vi "Roll Process.vi"() -> ()   [LabVIEW 2009]
uses:
  <vilib>/Utility/file.llb/Read From Spreadsheet File (string).vi
  <vilib>/Utility/file.llb/Write To Spreadsheet File (string).vi
panel:
  out "P 4":string[](array[string])
  out "P 3":string[](array[string])
  out "P 2":string[](array[string])
  out "P 1":string[](array[string])
  out "L 4":string[](array[string])
  out "L 3":string[](array[string])
  out "L 2":string[](array[string])
  out "L 1":string[](array[string])
  out "Cool Down Laps":string[](array[string])
  out "Warm Up Laps":string[](array[string])
  out "Cycle":string[](array[string])
  out "Length":string[](array[string])
  out "Chamber":string[](array[string])
  out "Value":string[][](array[string])
  in  "New Recipe":bool
  in  "Recipe Name":string
  in  "Save Recipe File":bool
  in  "Load Recipe File":bool
  in  "Recipe Table":string[][](table)
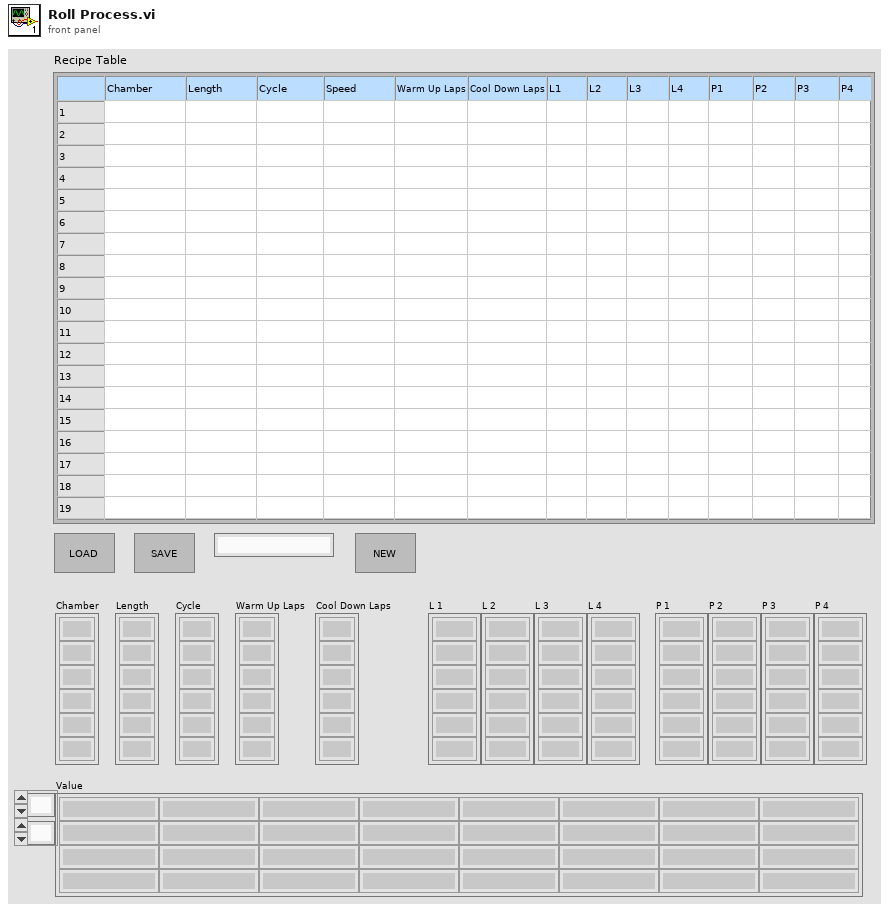
[diagram p1: front panel]
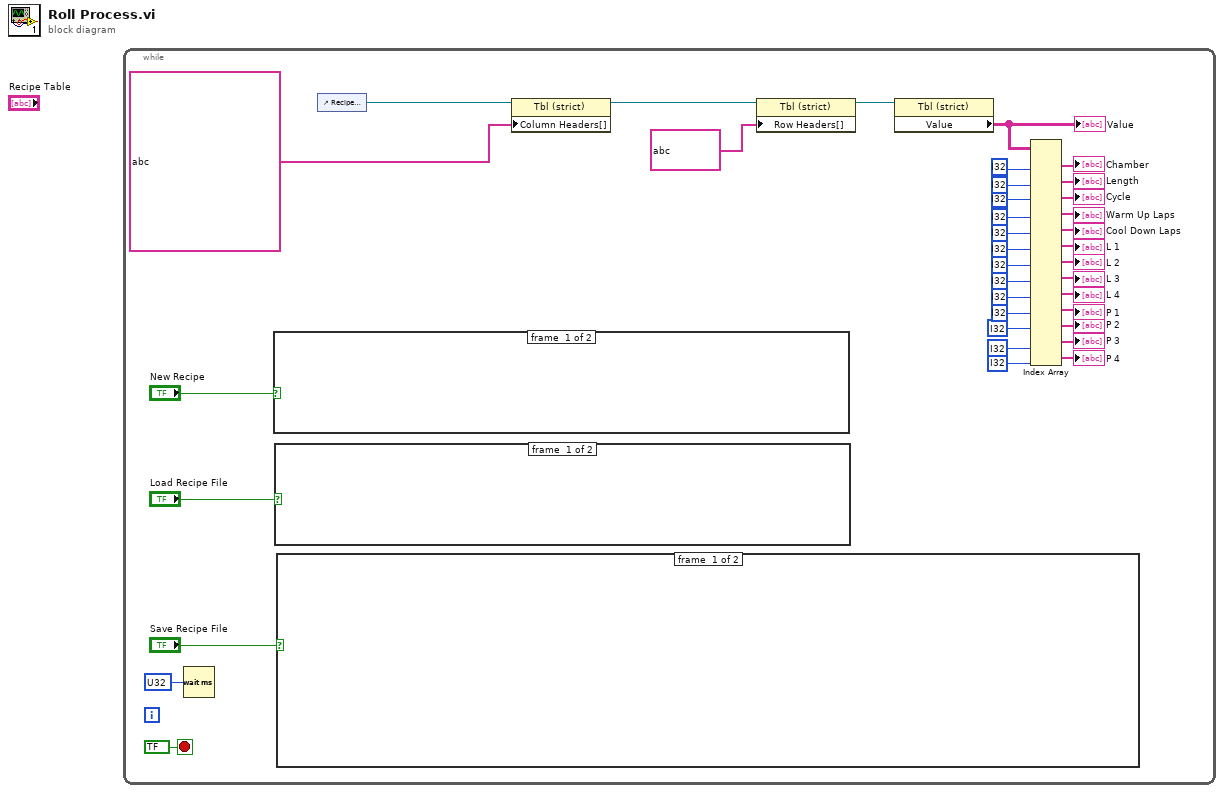
[diagram p0: block diagram]
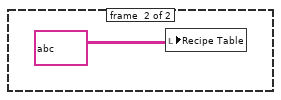
[diagram p2: hidden frame]
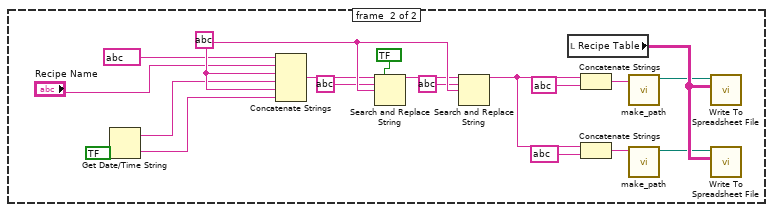
[diagram p3: hidden frame]
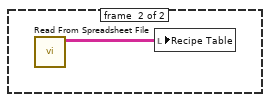
[diagram p4: hidden frame]
diagram:
  n1 = while {
    stop <- bool ? stop-if-true
    n2 = Wait (ms)(milliseconds to wait=u32 ?) -> ()  [unwired: 1 out]
    n3 = case shown="True" "New Recipe" {
      frame #0 {
      }
      frame #1 {
        n4 = local write "Recipe Table"(string[][] ? ("Row Header Strings[]")) -> ()
      }
    }
    n5 = case shown="True" "Load Recipe File" {
      frame #0 {
      }
      frame #1 {
        n6 = call-poly <vilib>:"Read From Spreadsheet File.vi"() -> ("all rows"=w58:string[][])  [unwired: 7 in, 4 out]
        n7 = local write "Recipe Table"(w58) -> ()
      }
    }
    n8 = case shown="True" "Save Recipe File" {
      frame #0 {
      }
      frame #1 {
        w49 = string ? ("string")
        n9 = Get Date/Time String(want seconds? (F)=bool ?) -> (date string=w42:string, time string=w43:string)  [unwired: 2 in]
        n10 = Concatenate Strings(string ? ("file_name"), "Recipe Name", w49, w42, w49, w43) -> (w44:string)
        n11 = Search and Replace String(replace all?=bool ? ("replace all? (F)"), input string=w44, search string=string ?, replace string=w49) -> (result string=w47:string)  [unwired: 4 in, 3 out]
        n12 = Search and Replace String(input string=w47, search string=string ?, replace string=w49) -> (result string=w51:string)  [unwired: 5 in, 3 out]
        n13 = local read "Recipe Table"() -> (w57:string[][])
        n14 = Concatenate Strings(w51, string ? ("string")) -> (w53:string)
        n15 = Concatenate Strings(w51, string ? ("string")) -> (w54:string)
        n16 = call "make_path.vi"("file_name"=w53) -> ("file path"=w55:path)  [unwired: 10 in]
        n17 = call "make_path.vi"("file_name"=w54) -> ("file path"=w56:path)  [unwired: 10 in]
        n18 = call-poly <vilib>:"Write To Spreadsheet File.vi"("2D data"=w57, "file path (dialog if empty)"=w55) -> ()  [unwired: 6 in, 1 out]
        n19 = call-poly <vilib>:"Write To Spreadsheet File.vi"("2D data"=w57, "file path (dialog if empty)"=w56) -> ()  [unwired: 6 in, 1 out]
      }
    }
    n20 = control-ref of="Recipe Table"() -> (w29:refnum<vi>)
    n21 = property class="Tbl (strict)"(reference=w29, "Column Headers[]"=string[] ? ("Column Header Strings[]")) -> (reference out=w37:refnum<vi>)  [unwired: 1 in, 1 out]
    n22 = property class="Tbl (strict)"(reference=w37, "Row Headers[]"=string[] ? ("Row Header Strings[]")) -> (reference out=w28:refnum<vi>)  [unwired: 1 in, 1 out]
    n23 = property class="Tbl (strict)"(reference=w28) -> ("Value"=w27:string[][])  [unwired: 1 in, 2 out]
    "Value" <- w27
    n24 = Index Array(array=w27, index (col) #1=i32 ? ("length"), index (col) #2=i32 ? ("index (col)"), index (col) #3=i32 ? ("index (col)"), index (col) #4=i32 ? ("index (col)"), index (col) #5=i32 ? ("index (col)"), index (col) #6=i32 ? ("index (col)"), index (col) #7=i32 ? ("index (col)"), index (col) #8=i32 ? ("index (col)"), index (col) #9=i32 ? ("index (col)"), index (col) #10=i32 ? ("index (col)"), index (col) #11=i32 ? ("index (col)"), index (col) #12=i32 ? ("index (col)"), index (col) #13=i32 ? ("index (col)")) -> (element #1=→"Chamber":string[], element #2=→"Length":string[], element #3=→"Cycle":string[], element #4=→"Warm Up Laps":string[], element #5=→"Cool Down Laps":string[], element #6=→"L 1":string[], element #7=→"L 2":string[], element #8=→"L 3":string[], element #9=→"L 4":string[], element #10=→"P 1":string[], element #11=→"P 2":string[], element #12=→"P 3":string[], element #13=→"P 4":string[])  [unwired: 13 in]
  }
